vi "Introspection Core.vi"(8 "error in (no error)":errorcluster, 11 "CS++BaseActor in":refnum<class "CS++BaseActor.lvclass">) -> (0 "error out":errorcluster, 2 "CS++Messages":refnum<class "Message.lvclass">[](array[class]), 3 "CS++BaseActor out":refnum<class "CS++BaseActor.lvclass">)   [LabVIEW 2014, in "CS++BaseActor.lvlib" / "CS++BaseActor.lvclass"]
doc: "This vi delivers a list with all messages this actor reacts to. \n\nNote that all inherited classes have to overwrite it."
uses:
  CS++BaseActor.lvclass
  CS++BaseActor Messages/After Launch Init Msg/After Launch Init Msg.lvclass
  CS++BaseActor Messages/Launch Associated GUI Msg/Launch Associated GUI Msg.lvclass
  CS++BaseActor Messages/Open Actor Core FP Msg/Open Actor Core FP Msg.lvclass
  <vilib>/ActorFramework/Message/Message.lvclass
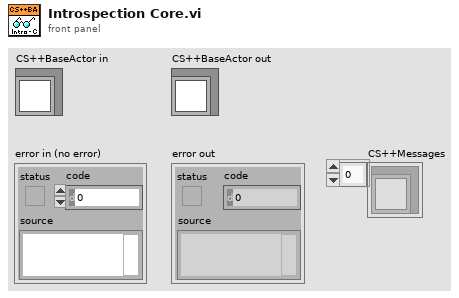
[diagram p1: front panel]
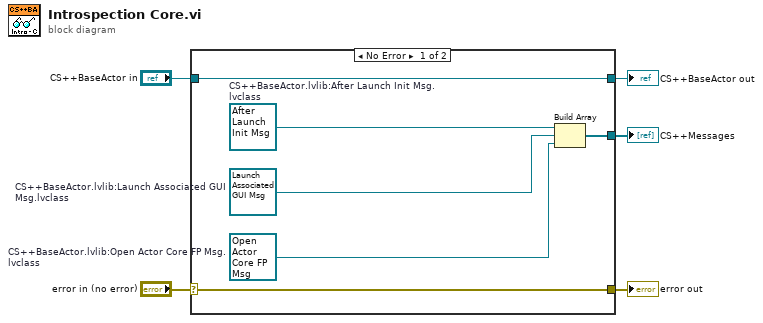
[diagram p0: block diagram]
diagram:
  n1 = case shown="No Error" "error in (no error)" {
    selector: "error in (no error)" -> [w10 w13]
    tunnel: [w10 w13] -> w4
    tunnel: [w11 w12] -> w2
    tunnel: "CS++BaseActor in" -> [w11 w12]
    tunnel: [w6 _] -> w1
    frame No Error {
      w7 = refnum<class "Open Actor Core FP Msg.lvclass"> refnum  # CS++BaseActor.lvlib:Open Actor Core FP Msg.lvclass
      w8 = refnum<class "Launch Associated GUI Msg.lvclass"> refnum  # CS++BaseActor.lvlib:Launch Associated GUI Msg.lvclass
      w9 = refnum<class "After Launch Init Msg.lvclass"> refnum  # CS++BaseActor.lvlib:After Launch Init Msg.lvclass
      n2 = Build Array(w9, w8, w7) -> (w6:refnum<class "Message.lvclass">[])
    }
    frame Error {
    }
  }
  "error out" <- w4
  "CS++BaseActor out" <- w2
  "CS++Messages" <- w1
